vi "_Read.vi"(8 "error in (no error)":errorcluster, 11 "Fluke Calibrator in":refnum<class "Fluke Calibrator.lvclass">) -> (0 "error out":errorcluster, 2 "X array":T1, 3 "Fluke Calibrator out":refnum<class "Fluke Calibrator.lvclass">)   [LabVIEW 2017, in "Fluke Calibrator.lvclass"]
doc: "(Protected, Dynamic, Pure Virtual/Abstract) Perform a measurement and return one or more channels of data. Outsiders should not call this method, but instead the public \"Read Data.vi\"."
uses:
  Fluke Calibrator.lvclass
  Utility Classes/Readable/Readable.lvclass
  Utility Classes/Readable/X.ctl
  Utility Classes/Readable/X array.ctl
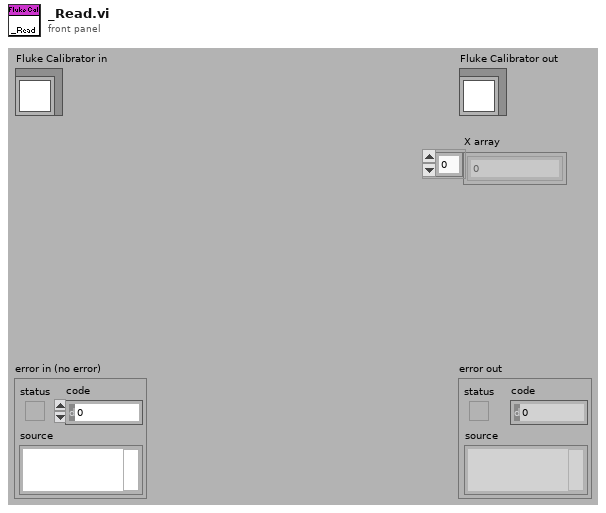
[diagram p1: front panel]
types:
  T1 = typedef "Readable.lvclass/X array.ctl" = T2[]
  T2 = typedef "Readable.lvclass/X.ctl" = dbl
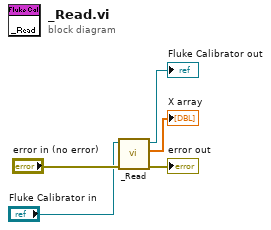
[diagram p0: block diagram]
diagram:
  n1 = call-parent "_Read.vi"("error in (no error)"="error in (no error)", "Readable in"="Fluke Calibrator in") -> ("error out"=→"error out":errorcluster, "X array"=→"X array":T1, "Readable out"=→"Fluke Calibrator out":refnum<class "Fluke Calibrator.lvclass">)  [unwired: 7 in]
